vi "emi_Send S&E Notefication.vi"(1 "Note(\"\")":string, 2 "Send(T)":bool=TRUE, 5 "Loop ID in(No ID)":u16=9999, 9 "error in (no error)":errorcluster, 12 "Loc Sub ID/Note ID":u16, 13 "Elevated priority":bool) -> (6 "Loop ID out":u16, 10 "error out":errorcluster)   [LabVIEW 2011]
doc: "Send a Noteficeaiton on the S&E Bus"
uses:
  Private/_emi_ S&E Message.ctl
  Private/_emi_ S&E Message type.ctl
  Private/_emi_GFV System ID.vi
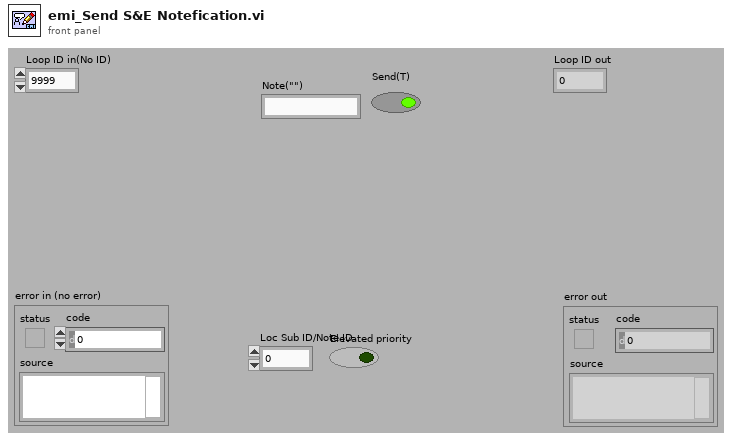
[diagram p1: front panel]
types:
  T1 = typedef "_emi_ S&E Message type.ctl" = enum16{"Error/Warning", "Note", "Debug", "Event", "Alarm Analog", "Alarm Digital", "Annotation"}
  T2 = typedef "_emi_ S&E Message.ctl" = cluster{"Type":T1, "Originate time":dbl, "System":u8, "Loop":u16, "Sub ID":u16, "Elevated priority":bool, "E&S Message content":variant}
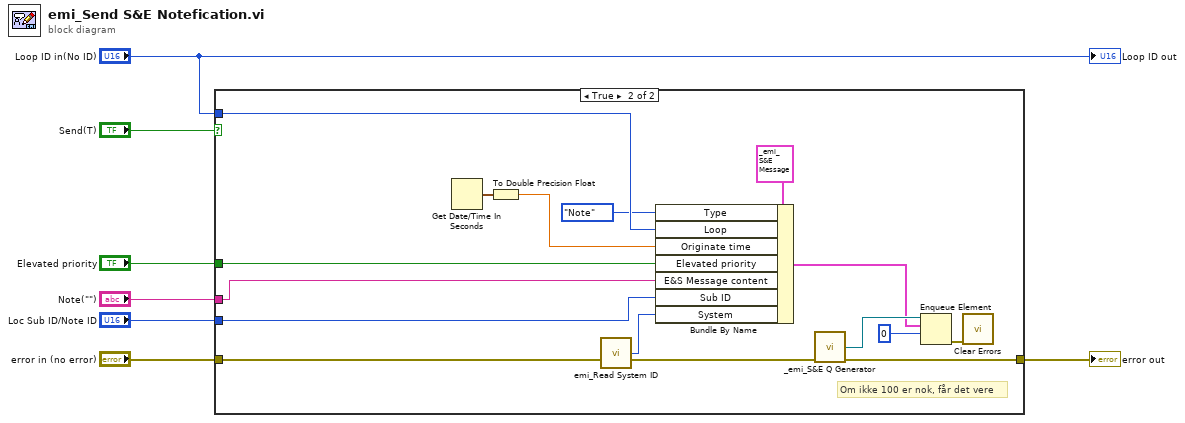
[diagram p0: block diagram]
diagram:
  n1 = case shown="True" "Send(T)" {
    tunnel: "Loop ID in(No ID)" -> [_ w20]
    tunnel: "Elevated priority" -> [_ w21]
    tunnel: "error in (no error)" -> [w8 w12]
    tunnel: [w8 w18] -> w4
    tunnel: "Note(\"\")" -> [_ w9]
    tunnel: "Loc Sub ID/Note ID" -> [_ w14]
    frame False {
    }
    frame True {
      # "Om ikke 100 er nok, får det vere"
      n2 = Get Date/Time In Seconds() -> (seconds since 1Jan1904=w22:timestamp)
      n3 = To Double Precision Float(number=w22) -> (double precision float=w23:dbl)
      n4 = call "emi_Read System ID.vi"("error in (no error)"=w12) -> ("System ID"=w10:u8, "error out"=w11:errorcluster)  [unwired: 13 in]
      n5 = Bundle By Name(cluster=T2 {"Type"=enum."Error/Warning", "Originate time"=0.0, "System"=0, "Loop"=0, "Sub ID"=0, "Elevated priority"=FALSE, "E&S Message content"=variant} ("E&S Message"), "Type"=_emi__S&E_Message_type."Note", "Loop"=w20, "Originate time"=w23, "Elevated priority"=w21, "E&S Message content"=w9, "Sub ID"=w14, "System"=w10) -> (w16:T2)
      n6 = call "_emi_S&E Q Generator.vi"("error in (no error)"=w11) -> ("E&S Message Q"=w17:refnum<queue>, "error out"=w18:errorcluster)  [unwired: 13 in]
      n7 = Enqueue Element(queue=w17, element=w16, timeout in ms (-1)=0) -> (error out=w13:errorcluster)  [unwired: 1 in, 2 out]
      n8 = call <vilib>:"Clear Errors.vi"("error in (no error)"=w13) -> ()  [unwired: 6 in, 1 out]
    }
  }
  "error out" <- w4
  "Loop ID out" <- "Loop ID in(No ID)"
